vi "Jeffress_model_v003.vi"() -> ()   [LabVIEW 2019]
panel:
  out "Elapsed time 2":dbl
  out "new picture":picture
  out "Left - Right":dbl
  out "Elapsed time 1":dbl caption="Get Start Time (s)"
  in  "stop":bool
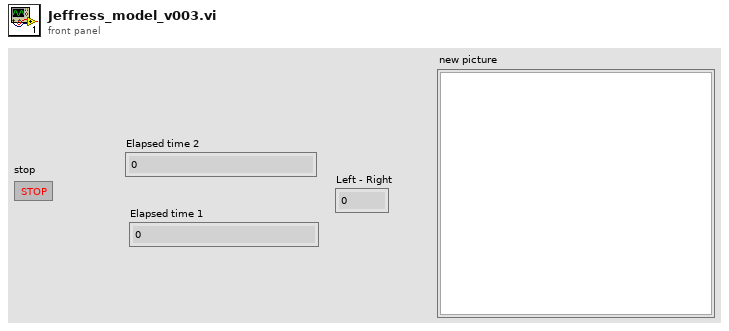
[diagram p1: front panel]
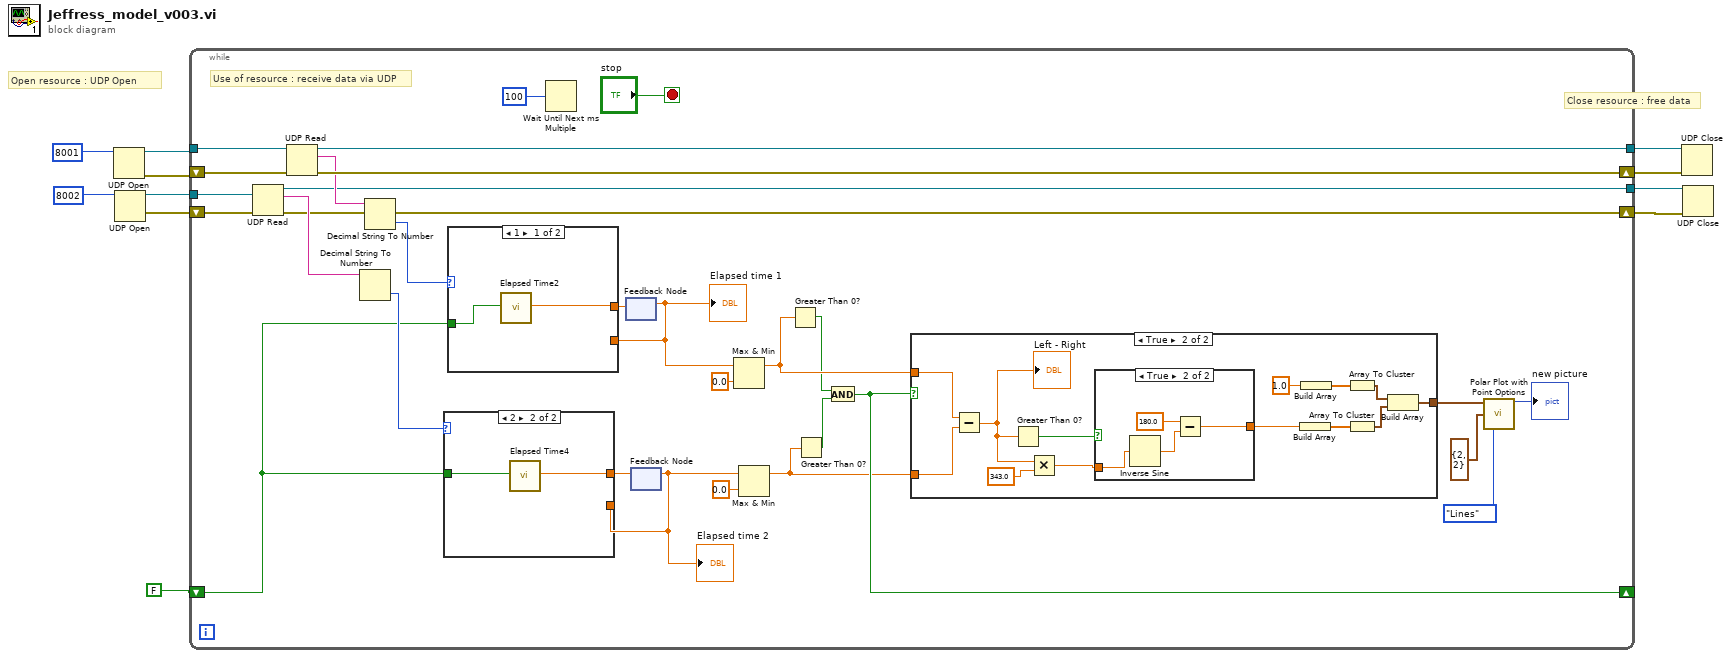
[diagram p0: block diagram]
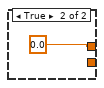
[diagram p3: hidden frame]
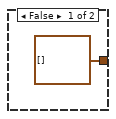
[diagram p4: hidden frame]
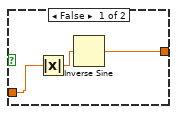
[diagram p5: hidden frame]
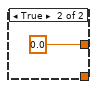
[diagram p7: hidden frame]
diagram:
  # "Close resource : free data"
  # "Open resource : UDP Open"
  n1 = UDP Open(11:u16 8001) -> (port=w9:refnum<k16>, 0:w11:errorcluster)  [unwired: 4 in, 1 out]
  n2 = UDP Open(11:u16 8002) -> (port=w4:refnum<k16>, 0:w3:errorcluster)  [unwired: 4 in, 1 out]
  n3 = while {
    tunnel: w9 -> [w37]
    tunnel: [w36] -> w8
    shift-right: [w39] -> w10
    shift-left: w11 -> [w38]
    shift-right: [w32] -> _
    shift-left: FALSE -> [w19]
    tunnel: w4 -> [w22]
    shift-right: [w12] -> w2
    shift-left: w3 -> [w21]
    tunnel: [w13] -> w1
    stop <- "stop" stop-if-true
    # "Use of resource : receive data via UDP"
    n4 = UDP Read(connection ID=w22, 8:w21) -> (data out=w23:string, error out=w12:errorcluster, 3:w13:refnum<k16>)  [unwired: 2 in, 2 out]
    n5 = UDP Read(connection ID=w37, 8:w38) -> (data out=w24:string, error out=w39:errorcluster, 3:w36:refnum<k16>)  [unwired: 2 in, 2 out]
    n6 = Decimal String To Number(string=w23) -> (number=w20:i32)  [unwired: 2 in, 1 out]
    n7 = Decimal String To Number(string=w24) -> (number=w25:i32)  [unwired: 2 in, 1 out]
    n8 = Wait Until Next ms Multiple(millisecond multiple=u32 100) -> ()  [unwired: 1 out]
    n9 = feedback #1() -> (w15:dbl)  [unwired: 1 in]
    "Elapsed time 1" <- w15
    n10 = case shown="1" w25 {
      tunnel: w19 -> [w71 w74]
      tunnel: [w70 w73] -> w18
      tunnel: w15 -> [_ w72]
      frame 1 {
        n11 = call "Elapsed Time2"("Reset"=w71) -> ("Elapsed Time (s)"=w70:dbl)  [unwired: 11 in, 7 out]
      }
      frame Default {
        n12 = case shown="False" w74 {
          tunnel: [w75 0.0] -> w73
          tunnel: w72 -> [w75 _]
          frame False {
          }
          frame True {
          }
        }
      }
    }
    n13 = feedback-in #1(w18) -> ()
    n14 = feedback #2() -> (w16:dbl)  [unwired: 1 in]
    "Elapsed time 2" <- w16
    n15 = case shown="2" w20 {
      tunnel: [w43 w48] -> w17
      tunnel: w19 -> [w44 w47]
      tunnel: w16 -> [w42 _]
      frame Default {
        n16 = case shown="False" w44 {
          tunnel: [w45 0.0] -> w43
          tunnel: w42 -> [w45 _]
          frame False {
          }
          frame True {
          }
        }
      }
      frame 2 {
        n17 = call "Elapsed Time4"("Reset"=w47) -> ("Elapsed Time (s)"=w48:dbl)  [unwired: 11 in, 7 out]
      }
    }
    n18 = feedback-in #2(w17) -> ()
    n19 = Max & Min(x=w15, y=0.0) -> (max(x,y)=w30:dbl)  [unwired: 1 out]
    n20 = Max & Min(x=w16, y=0.0) -> (max(x,y)=w31:dbl)  [unwired: 1 out]
    n21 = Greater Than 0?(x=w30) -> (x > 0?=w14:bool)
    n22 = Greater Than 0?(x=w31) -> (x > 0?=w33:bool)
    n23 = And(x=w14, y=w33) -> (x .and. y?=w32:bool)
    n24 = case shown="True" w32 {
      tunnel: w30 -> [_ w61]
      tunnel: w31 -> [_ w62]
      tunnel: [cluster{"[0]":dbl, "[1]":dbl}[] [] w53] -> w29
      frame False {
      }
      frame True {
        n25 = Subtract(x=w61, y=w62) -> (x-y=w50:dbl)
        "Left - Right" <- w50
        n26 = Greater Than 0?(x=w50) -> (x > 0?=w60:bool)
        n27 = Multiply(x=w50, y=343.0) -> (x*y=w51:dbl)
        n28 = case shown="True" w60 {
          tunnel: w51 -> [w63 w69]
          tunnel: [w65 w66] -> w56
          frame False {
            n29 = Absolute Value(x=w63) -> (abs(x)=w64:dbl)
            n30 = Inverse Sine(1:w64) -> (0:w65:dbl)
          }
          frame True {
            n31 = Inverse Sine(1:w69) -> (0:w68:dbl)
            n32 = Subtract(x=180.0, y=w68) -> (x-y=w66:dbl)
          }
        }
        n33 = Build Array(w56) -> (w57:dbl[])
        n34 = Build Array(1.0 ("element")) -> (w58:dbl[])
        n35 = Array To Cluster(array=w58) -> (cluster=w54:cluster{"[0]":dbl, "[1]":dbl})
        n36 = Array To Cluster(array=w57) -> (cluster=w55:cluster{"[0]":dbl, "[1]":dbl})
        n37 = Build Array(w54, w55) -> (w53:cluster{"[0]":dbl, "[1]":dbl}[])
      }
    }
    n38 = call <vilib>:"Polar Plot with Point Options.vi"("data array [mag, phase (deg)]"=w29, "top left point(0, 0)"=cluster{"x":i16, "y":i16} {"x"=2, "y"=2}, "Lines/Points"=enum16{"Lines", "Points"}."Lines") -> ("new picture"=→"new picture":picture)  [unwired: 12 in]
  }
  n39 = UDP Close(connection ID=w8, 8:w10) -> ()  [unwired: 2 out]
  n40 = UDP Close(connection ID=w1, 8:w2) -> ()  [unwired: 2 out]
